vi "Open.vi"(8 "Error In":errorcluster, 10 "Enable Gestures? (T)":bool=TRUE) -> (0 "Error Out":errorcluster, 3 "Leap Handle":T1)   [LabVIEW 2011, in "LVH-Leap.lvlib"]
doc: "Leap Open allows you to open a connection to the Leap Motion Controller with the option of having gestures enabled. When <b>Enable Gestures?</b> is true, all available gestures are turned on including Circle, Swipe, Screen Tap, and Key Tap detection.\n\nIf gestures are not being used then set <b>Enable Gestures?</b> to false to reduce the amount of resource utilization required by the Leap Motion for processing gestures."
uses:
  LVH-Leap.lvlib
  Private/Type Defs/Leap Handle.ctl
  C:/github/labviewhacker/LVH-Leap/LabVIEW/vi.lib/LabVIEW Hacker/Leap/Private/Libs/LeapCSharp.NET3.5.dll
  Private/Libs/LeapCSharp.NET3.5.dll
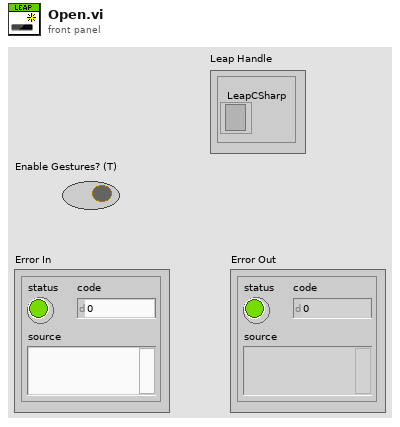
[diagram p1: front panel]
types:
  T1 = typedef "LVH-Leap.lvlib/Leap Handle.ctl" = cluster{"LeapCSharp":refnum<k24>}
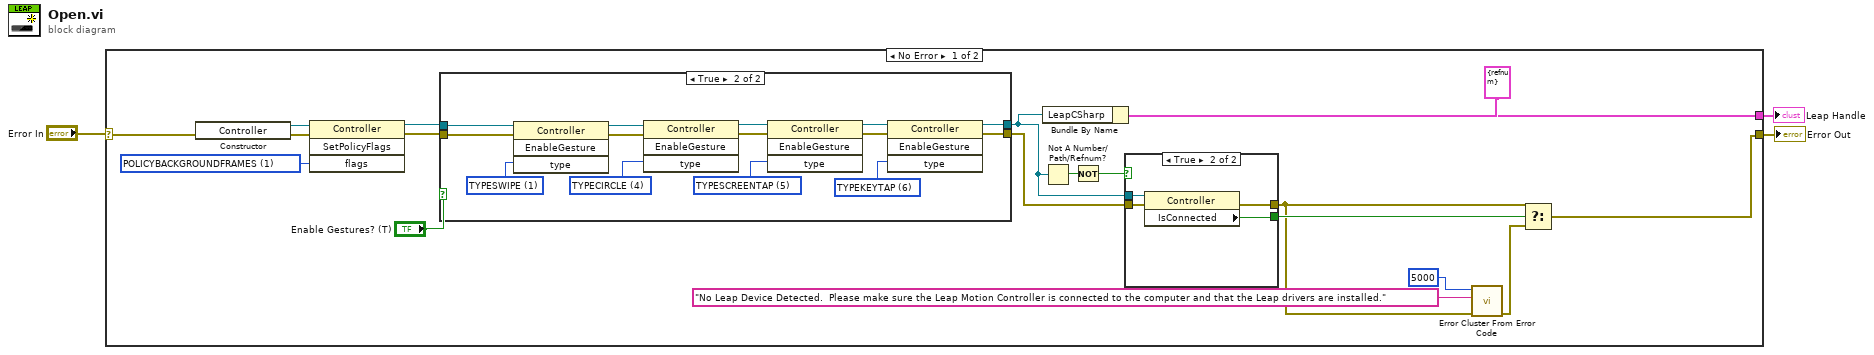
[diagram p0: block diagram]
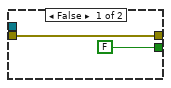
[diagram p2: hidden frame]
diagram:
  n1 = case shown="No Error" "Error In" {
    selector: "Error In" -> [w22 w45]
    tunnel: [w5 w45] -> w1
    tunnel: [w20 _] -> w3
    frame No Error {
      w14 = 1 items=["POLICYDEFAULT", "POLICYBACKGROUNDFRAMES"] ("flags")
      n2 = constructor class="Controller"(error in=w22) -> (reference out=w15:refnum<k24>, error out=w18:errorcluster)  [unwired: 2 in, 1 out]
      n3 = invoke class="Controller" method="SetPolicyFlags"(reference=w15, error in=w18, "flags"=w14) -> (reference out=w16:refnum<k24>, error out=w17:errorcluster)  [unwired: 1 in, 2 out]
      n4 = case shown="True" "Enable Gestures? (T)" {
        tunnel: w16 -> [w29 w44]
        tunnel: w17 -> [w30 w43]
        tunnel: [w30 w42] -> w10
        tunnel: [w29 w41] -> w11
        frame False {
        }
        frame True {
          w33 = 6 items=["TYPESWIPE"=1, "TYPECIRCLE"=4, "TYPESCREENTAP"=5, "TYPEKEYTAP"=6, "TYPEINVALID"=-1] ("type")
          w36 = 5 items=["TYPESWIPE"=1, "TYPECIRCLE"=4, "TYPESCREENTAP"=5, "TYPEKEYTAP"=6, "TYPEINVALID"=-1] ("type")
          w37 = 4 items=["TYPESWIPE"=1, "TYPECIRCLE"=4, "TYPESCREENTAP"=5, "TYPEKEYTAP"=6, "TYPEINVALID"=-1] ("type")
          w40 = 1 items=["TYPESWIPE"=1, "TYPECIRCLE"=4, "TYPESCREENTAP"=5, "TYPEKEYTAP"=6, "TYPEINVALID"=-1] ("type")
          n5 = invoke class="Controller" method="EnableGesture"(reference=w44, error in=w43, "type"=w40) -> (reference out=w39:refnum<k24>, error out=w38:errorcluster)  [unwired: 1 in, 2 out]
          n6 = invoke class="Controller" method="EnableGesture"(reference=w39, error in=w38, "type"=w37) -> (reference out=w35:refnum<k24>, error out=w34:errorcluster)  [unwired: 1 in, 2 out]
          n7 = invoke class="Controller" method="EnableGesture"(reference=w35, error in=w34, "type"=w36) -> (reference out=w31:refnum<k24>, error out=w32:errorcluster)  [unwired: 1 in, 2 out]
          n8 = invoke class="Controller" method="EnableGesture"(reference=w31, error in=w32, "type"=w33) -> (reference out=w41:refnum<k24>, error out=w42:errorcluster)  [unwired: 1 in, 2 out]
        }
      }
      n9 = Bundle By Name(cluster=T1 {"LeapCSharp"=refnum} ("LeapController"), "LeapCSharp"=w11) -> (w20:T1)
      n10 = Not A Number/Path/Refnum?(number/path/refnum=w11) -> (NaN/Path/Refnum?=w13:bool)
      n11 = Not(x=w13) -> (.not. x?=w12:bool)
      n12 = case shown="True" w12 {
        tunnel: w11 -> [_ w28]
        tunnel: w10 -> [w23 w27]
        tunnel: [FALSE ("IsConnected") w26] -> w9
        tunnel: [w23 w25] -> w4
        frame False {
        }
        frame True {
          n13 = property class="Controller"(reference=w28, error in=w27) -> (error out=w25:errorcluster, "IsConnected"=w26:bool)  [unwired: 1 out]
        }
      }
      n14 = call <vilib>:"Error Cluster From Error Code.vi"("error in (no error)"=w4, "error message (\"\")"="No Leap Device Detected.  Please make sure the Leap Motion Controller is connected to the computer and that the Leap drivers are installed." ("error message (\"\")"), "error code (0)"=5000) -> ("error out"=w6:errorcluster)  [unwired: 6 in]
      n15 = Select(t=w4, s=w9, f=w6) -> (s? t:f=w5:errorcluster)
    }
    frame Error {
    }
  }
  "Leap Handle" <- w3
  "Error Out" <- w1
